vi "Image References.vi"(8 "error in":errorcluster) -> (0 "error out":errorcluster, 3 "Images":cluster{"Acquired Image":T1, "Display Image":T1})   [LabVIEW 2013]
uses:
  <vilib>/vision/Image Controls.llb/IMAQ Image.ctl
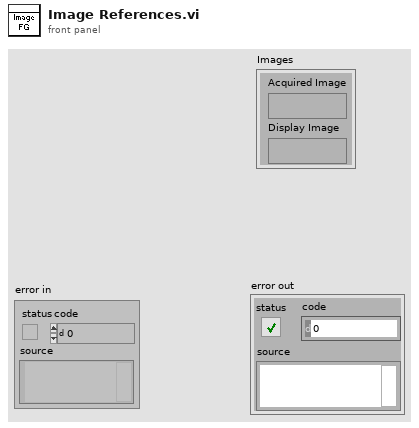
[diagram p1: front panel]
types:
  T1 = typedef "IMAQ Image.ctl" = refnum<image>
  T2 = typedef "Image Type" = u32
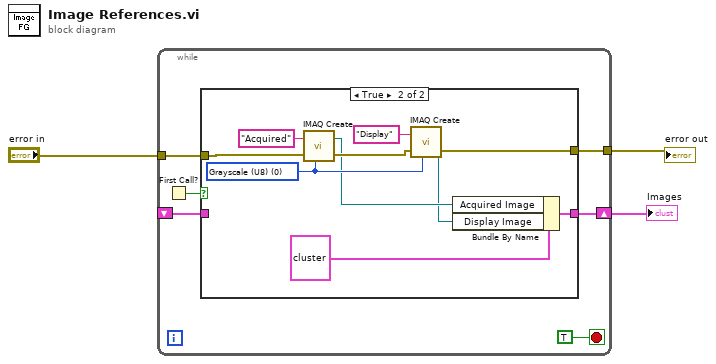
[diagram p0: block diagram]
diagram:
  n1 = while {
    tunnel: "error in" -> [w7]
    tunnel: [w6] -> w2
    shift-right: [w5] -> w1
    shift-left: _ -> [w4]
    stop <- TRUE stop-if-true
    n2 = First Call?() -> (First Call?: T/F=w8:bool)
    n3 = case shown="True" w8 {
      tunnel: w7 -> [w10 w19]
      tunnel: [w10 w17] -> w6
      tunnel: [w11 w12] -> w5
      tunnel: w4 -> [w11 _]
      frame False {
      }
      frame True {
        w16 = T2 0 items=["Grayscale (U8)", "Grayscale (I16)", "Grayscale (SGL)", "Complex (CSG)", "RGB (U32)", "HSL (U32)", "RGB (U64)", "Grayscale (U16)"] ("Image Type")
        n4 = call "IMAQ Create"("Image Name"="Acquired", "Image Type"=w16, "error in (no error)"=w19) -> ("New Image"=w14:T1, "error out"=w18:errorcluster)  [unwired: 2 in]
        n5 = call "IMAQ Create"("Image Name"="Display", "Image Type"=w16, "error in (no error)"=w18) -> ("New Image"=w13:T1, "error out"=w17:errorcluster)  [unwired: 2 in]
        n6 = Bundle By Name(cluster=cluster{"Acquired Image":T1, "Display Image":T1} {"Acquired Image"=refnum, "Display Image"=refnum} ("Images"), "Acquired Image"=w14, "Display Image"=w13) -> (w12:cluster{"Acquired Image":T1, "Display Image":T1})
      }
    }
  }
  "Images" <- w1
  "error out" <- w2
